vi "Reset Memory Blocks.vi"(0 "Memory Blocks In":T1) -> (2 "Memory Blocks Out":T1)   [LabVIEW 2016]
uses:
  Memory Block Channels.ctl
  MemoryBlocks.ctl
  <vilib>/Platform/TimedLoop/XDataNode/timing_clust.ctl
  <vilib>/Platform/TimedLoop/XDataNode/nitl_modes.ctl
  <vilib>/Platform/TimedLoop/XDataNode/wakeup.ctl
  <vilib>/rvi/Emulation/niFpgaSctlEmulationGetInTimedLoop.vi
  <vilib>/rvi/Emulation/niFpgaEmulationReportErrorSimple.vi
  <vilib>/rvi/Emulation/niFpgaGetClockAttributes.vi
  <vilib>/rvi/Emulation/niFpgaCriticalErrorInLSC.vi
  <vilib>/rvi/DataTransferAndStorage/Container/Common/niFpgaContainerExecOnDevCompGetState.vi
  <vilib>/rvi/Emulation/niFpgaEmulationIsFPGAContextNoSignature.vi
  <vilib>/rvi/DataTransferAndStorage/Container/Common/niFpgaContainerGetUniqueNameForEmu.vi
  <vilib>/rvi/Emulation/niFpgaProcessEmulError.vi
  <vilib>/rvi/errors/nirviReportUnexpectedCaseInternalError (U32).vi
  <vilib>/rvi/Memory/Memory_Emulation/niFpgaMemoryEmulationCacheClearOnFirstRun.vi
  <vilib>/rvi/Memory/Memory_Emulation/nirvimemoryEmulationManagerCache_MakeExclusive.vi
  <vilib>/rvi/Memory/Memory_Emulation/niFpgaMemoryEmulationValidateCache.vi
  <vilib>/rvi/Memory/Memory_Emulation/nirvimemoryEmulationManagerCache_InsertValue.vi
  <vilib>/Utility/error.llb/Clear Errors.vi
  <vilib>/rvi/Memory/Memory_Emulation/nirvimemoryEmulationManagerCache_ReleaseExclusive.vi
  <vilib>/rvi/Memory/Memory_Emulation/nirvimemoryEmulationManagerCache_GetValue.vi
  <vilib>/rvi/Memory/Memory_Emulation/nirvimemoryEmulationManagerCache_SetValue.vi
  <vilib>/rvi/Emulation/niFpgaSctlEmulationResourceMgr.vi
  <vilib>/Platform/TimedLoop/XDataNode/XDataNode.xnode
  <vilib>/rvi/DataTransferAndStorage/Container/XNode/niFpgaContainer.xnode
  <vilib>/rvi/Memory/Memory_Emulation/niFpgaMemoryEmulationRefIn.vi
  <vilib>/Platform/TimedLoop/XDataNode/XDNodeRunTimeDep.lvlib
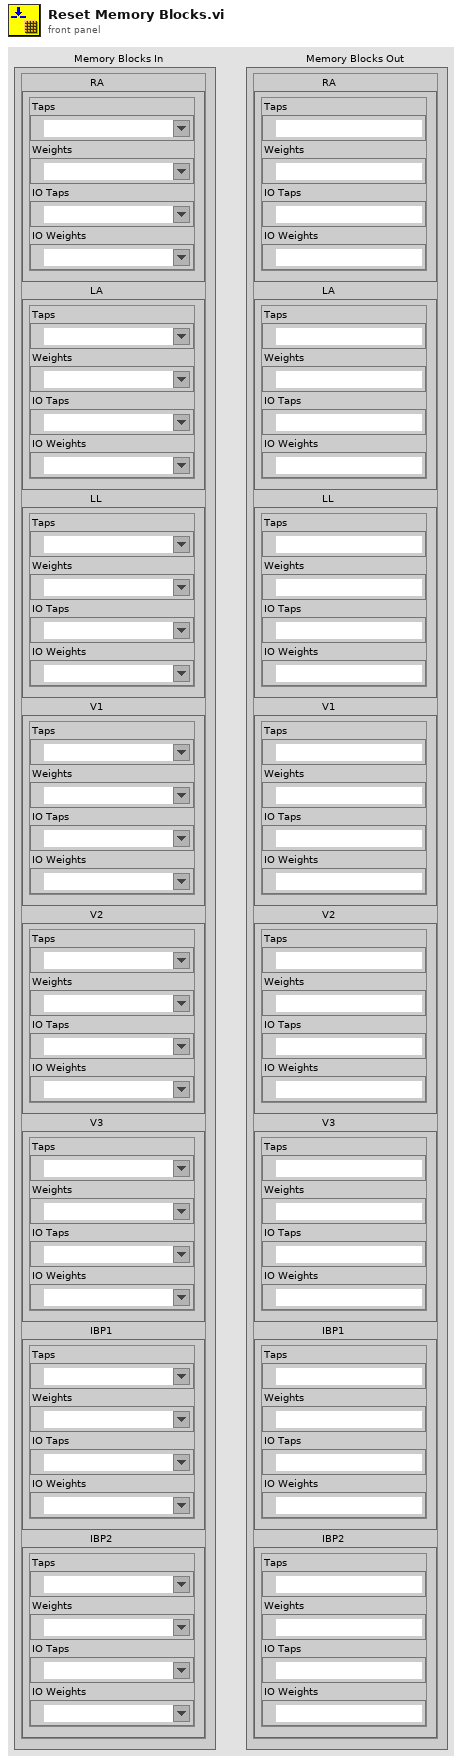
[diagram p1: front panel]
types:
  T1 = typedef "Memory Block Channels.ctl" = cluster{"RA":T2, "LA":T2, "LL":T2, "V1":T2, "V2":T2, "V3":T2, "IBP1":T2, "IBP2":T2}
  T2 = typedef "MemoryBlocks.ctl" = cluster{"Taps":refnum<k21>, "Weights":refnum<k21>, "IO Weights":refnum<k21>, "IO Taps":refnum<k21>}
  T3 = typedef "XDNodeRunTimeDep.lvlib/timing_clust.ctl" = cluster{"Expected End [f-1]":u64, "Actual End [f-1]":u64, "Finished Late? [f-1]":bool, "Expected End [i-1]":u64, "Actual End [i-1]":u64, "Finished Late? [i-1]":bool, "Expected Start [i]":u64, "Actual Start [i]":u64, "Expected Start [f]":u64, "Actual Start [f]":u64, "Source Name":string, "Structure Name":string, "Period":i64, "Deadline":i64, "Offset":i64, "Start":i64, "Priority":i32, "Timeout":i32, "Mode":T4, "Wakeup Reason":T5, "Error":errorcluster, "Source Type":string, "Secondary Source Type":string, "Global End Time":u64, "Global Start Time":u64, "Frame Duration":u64, "Iteration Duration":u64, "Assigned CPU":i32, "I/O Scan Engine Mode":u32}
  T4 = typedef "XDNodeRunTimeDep.lvlib/nitl_modes.ctl" = enum32{"No Change", "Process missed periods, maintain original phase", "Discard missed periods, maintain original phase", "Process missed periods, ignore original phase", "Discard missed periods, ignore original phase"}
  T5 = typedef "XDNodeRunTimeDep.lvlib/wakeup.ctl" = enum32{"Normal", "Aborted", "Asynchronous wakeup", "Timing source error", "Timed loop error", "Timeout"}
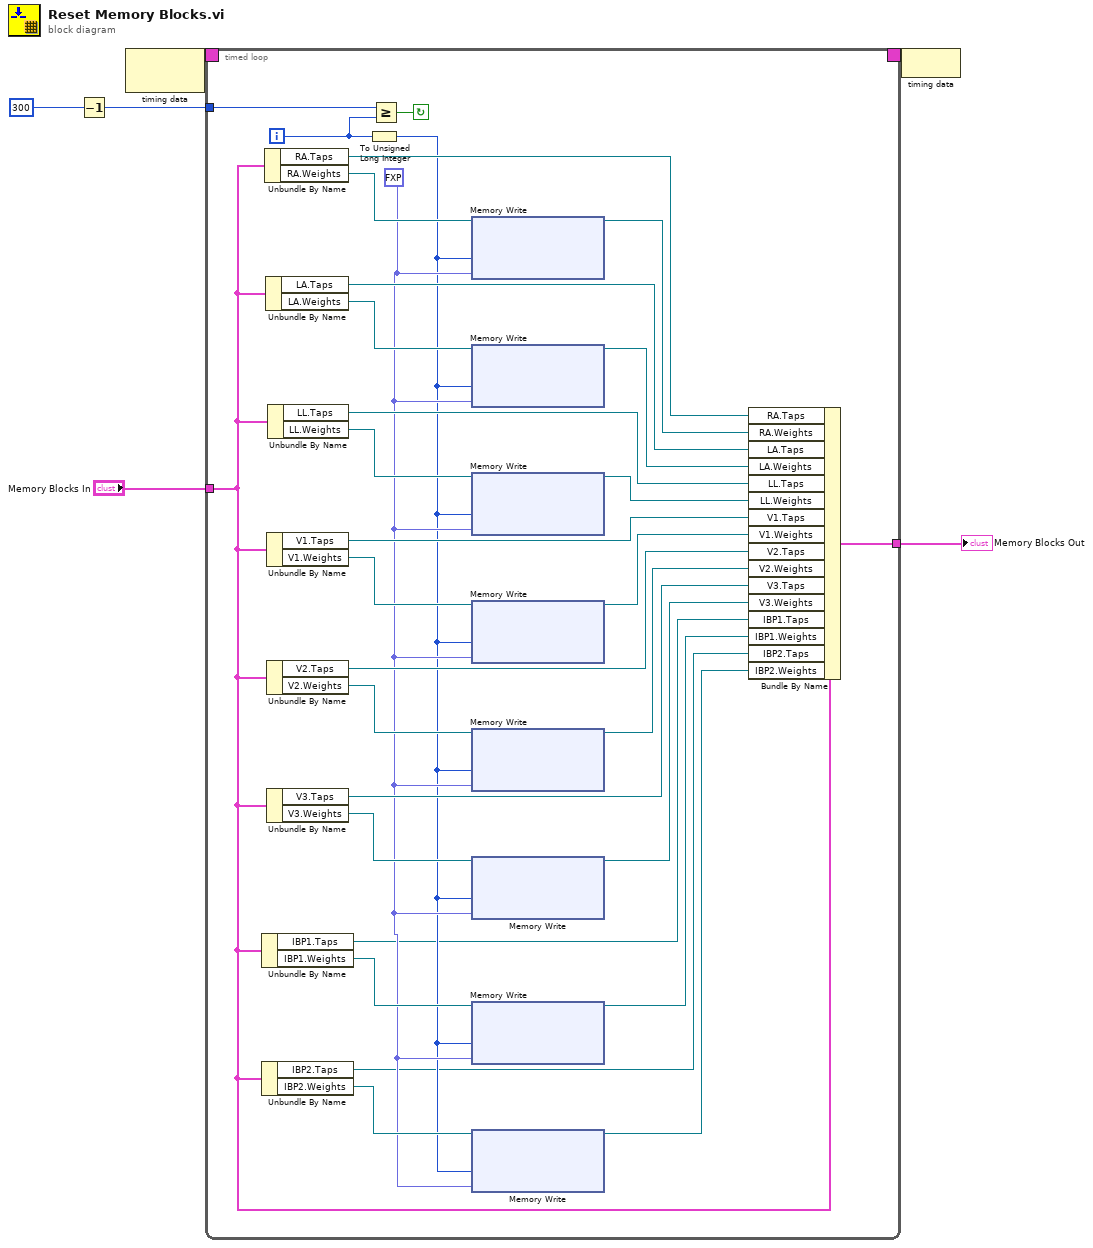
[diagram p0: block diagram]
diagram:
  n1 = Decrement(x=i16 300) -> (x-1=w2:i16)
  n2 = node-c288() -> (w6:T3)  [unwired: 1 in]
  n3 = timed-loop {
    timing: w6 -> [_]
    timing-out: [_] -> w5
    tunnel: w2 -> [w35]
    tunnel: "Memory Blocks In" -> [w11]
    tunnel: [w22] -> w4
    i -> [w36]
    stop <- w37 continue-if-true
    w13 = fxp<+/-,24,8> 0.0 ("Data")
    n4 = Unbundle By Name(w11) -> ("IBP1.Taps"=w10:refnum<k21>, "IBP1.Weights"=w14:refnum<k21>)
    n5 = Unbundle By Name(w11) -> ("IBP2.Taps"=w8:refnum<k21>, "IBP2.Weights"=w15:refnum<k21>)
    n6 = Unbundle By Name(w11) -> ("RA.Taps"=w16:refnum<k21>, "RA.Weights"=w34:refnum<k21>)
    n7 = Unbundle By Name(w11) -> ("LA.Taps"=w17:refnum<k21>, "LA.Weights"=w33:refnum<k21>)
    n8 = Unbundle By Name(w11) -> ("V1.Taps"=w19:refnum<k21>, "V1.Weights"=w31:refnum<k21>)
    n9 = Unbundle By Name(w11) -> ("V2.Taps"=w20:refnum<k21>, "V2.Weights"=w30:refnum<k21>)
    n10 = Unbundle By Name(w11) -> ("V3.Taps"=w21:refnum<k21>, "V3.Weights"=w29:refnum<k21>)
    n11 = Unbundle By Name(w11) -> ("LL.Taps"=w18:refnum<k21>, "LL.Weights"=w32:refnum<k21>)
    n12 = To Unsigned Long Integer(number=w36) -> (unsigned 32bit integer=w12:u32)
    n13 = Greater Or Equal?(x=w35, y=w36) -> (x >= y?=w37:bool)
    n14 = xnode ("Memory Write")("Address"=w12, "Data"=w13, "Memory In"=w34) -> ("Memory Out"=w26:refnum<k21>)
    n15 = xnode ("Memory Write")("Address"=w12, "Data"=w13, "Memory In"=w33) -> ("Memory Out"=w27:refnum<k21>)
    n16 = xnode ("Memory Write")("Address"=w12, "Data"=w13, "Memory In"=w32) -> ("Memory Out"=w28:refnum<k21>)
    n17 = xnode ("Memory Write")("Address"=w12, "Data"=w13, "Memory In"=w31) -> ("Memory Out"=w25:refnum<k21>)
    n18 = xnode ("Memory Write")("Address"=w12, "Data"=w13, "Memory In"=w30) -> ("Memory Out"=w24:refnum<k21>)
    n19 = xnode ("Memory Write")("Address"=w12, "Data"=w13, "Memory In"=w29) -> ("Memory Out"=w23:refnum<k21>)
    n20 = xnode ("Memory Write")("Address"=w12, "Data"=w13, "Memory In"=w14) -> ("Memory Out"=w9:refnum<k21>)
    n21 = xnode ("Memory Write")("Address"=w12, "Data"=w13, "Memory In"=w15) -> ("Memory Out"=w7:refnum<k21>)
    n22 = Bundle By Name(cluster=w11, "RA.Taps"=w16, "RA.Weights"=w26, "LA.Taps"=w17, "LA.Weights"=w27, "LL.Taps"=w18, "LL.Weights"=w28, "V1.Taps"=w19, "V1.Weights"=w25, "V2.Taps"=w20, "V2.Weights"=w24, "V3.Taps"=w21, "V3.Weights"=w23, "IBP1.Taps"=w10, "IBP1.Weights"=w9, "IBP2.Taps"=w8, "IBP2.Weights"=w7) -> (w22:T1)
  }
  "Memory Blocks Out" <- w4
  n23 = node-c288(w5) -> ()
